vi "bind.vi"(8 "error in (no error)":errorcluster, 9 "sin6_port":dbl, 10 "sin6_addr":string, 11 "tcp socket fd":i32) -> (0 "error out":errorcluster, 3 "success":u16)   [LabVIEW 2015]
panel:
  in  "sin6_flowinto":dbl
  in  "sin6_family":string
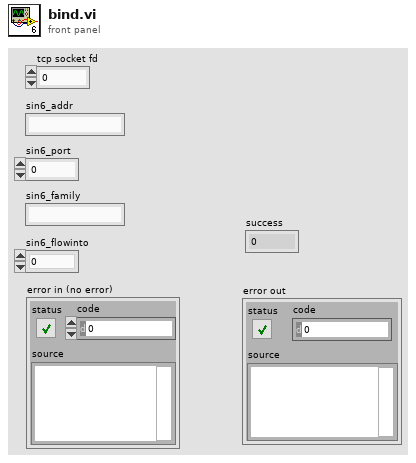
[diagram p1: front panel]
types:
  T1 = cluster{"sin6_family":string, "sin6_flowinto":dbl, "sin6_addr":string, "sin6_port":dbl}
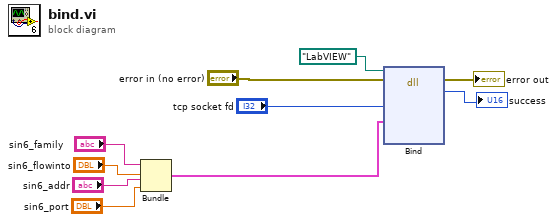
[diagram p0: block diagram]
diagram:
  n1 = Bundle("sin6_family"="sin6_family", "sin6_flowinto"="sin6_flowinto", "sin6_addr"="sin6_addr", "sin6_port"="sin6_port") -> (w1:T1)  [unwired: 1 in]
  n2 = dll-call lib="LabVIEW" fn="Bind"(path in=path "LabVIEW", error in="error in (no error)", "sockfd"="tcp socket fd", "sockaddr"=w1) -> (error out=→"error out":errorcluster, "success"=→"success":u16)  [unwired: 5 in, 1 out]
